vi "simulate_3d_spiral.vi"(8 "error in (no error)":errorcluster, 10 "open fp?":bool, 11 "TrajectoryMH100122AODRAPS in":refnum<class "TrajectoryMH100122AODRAPS.lvclass">) -> (0 "error out":errorcluster, 3 "TrajectoryMH100122AODRAPS out":refnum<class "TrajectoryMH100122AODRAPS.lvclass">)   [LabVIEW 2010, in "TrajectoryMH100122AODRAPS.lvclass"]
uses:
  TrajectoryMH100122AODRAPS.lvclass
  <vilib>/Math Plots/3D Math Plots/3D Scatter/3D Scatter XCtrl/3D Scatter.xctl
  <vilib>/Math Plots/3D Math Plots/3D Scatter/3D Scatter Datatype/Public/Plot Helper (Vector).vi
  <vilib>/Math Plots/3D Math Plots/3D Scatter/3D Scatter Datatype/3D Scatter Datatype.lvclass
panel:
  out "3D plot":refnum<class "3D Plot Datatype.lvclass">[](xcontrol)
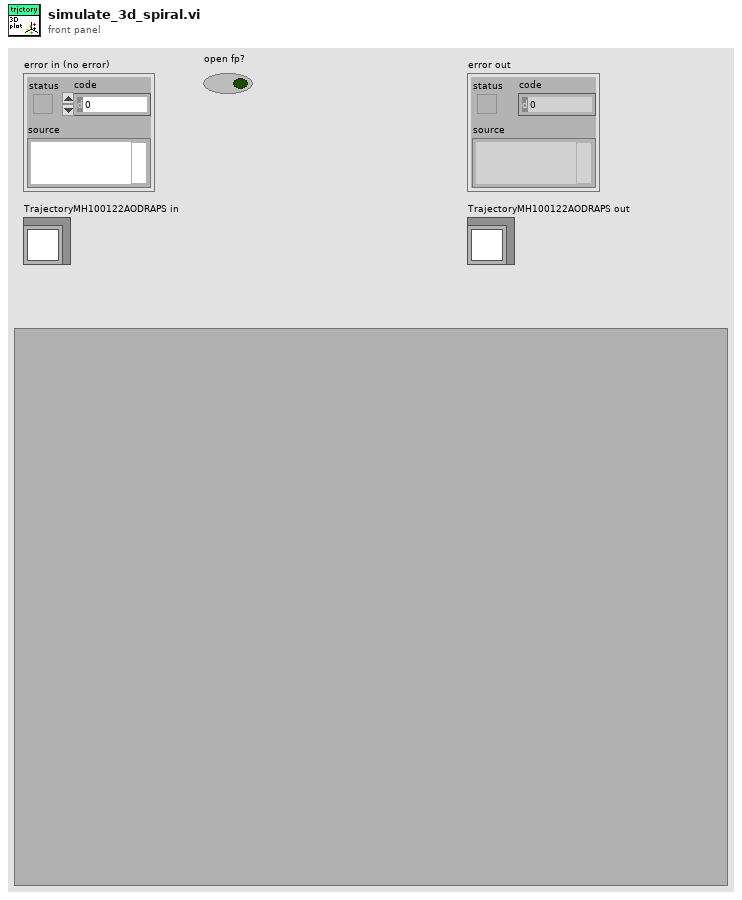
[diagram p1: front panel]
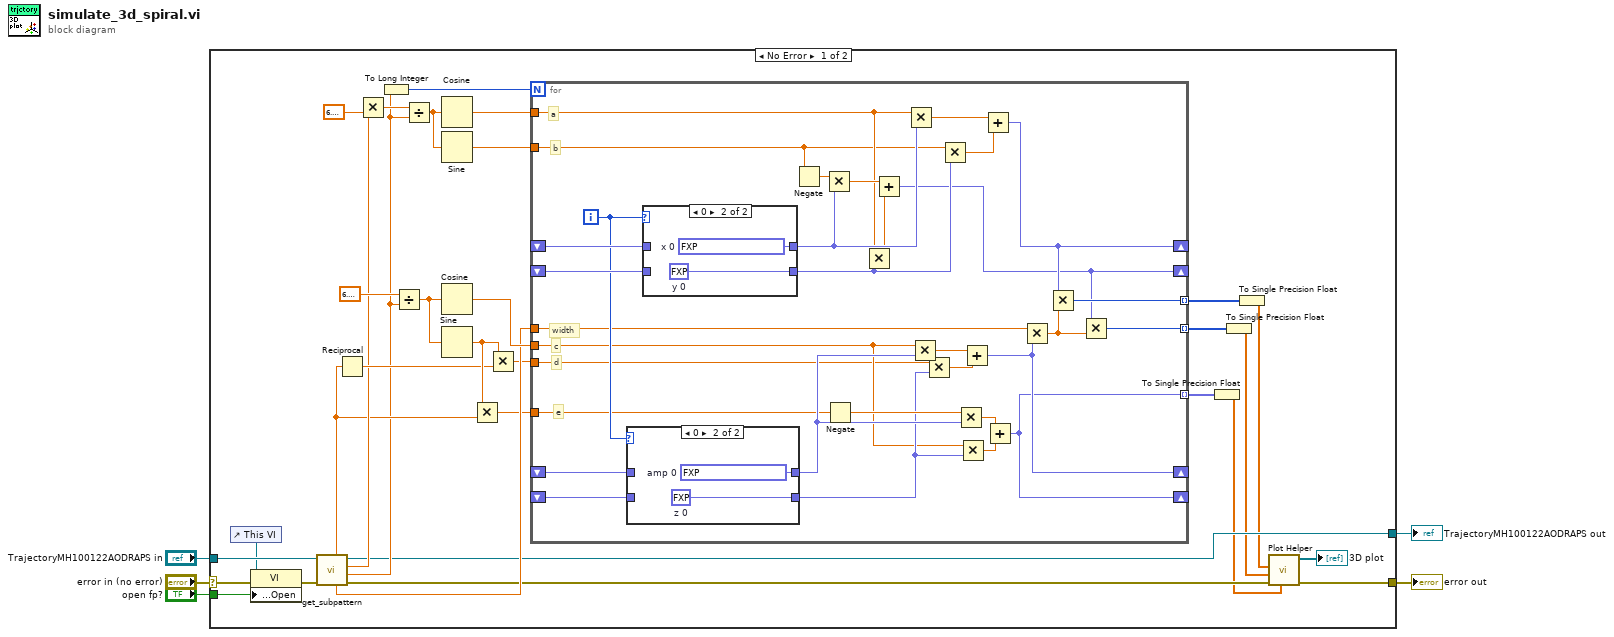
[diagram p0: block diagram]
diagram:
  n1 = case shown="No Error" "error in (no error)" {
    selector: "error in (no error)" -> [w9 w79]
    tunnel: [w18 w79] -> w4
    tunnel: [w17 w78] -> w2
    tunnel: "TrajectoryMH100122AODRAPS in" -> [w37 w78]
    tunnel: "open fp?" -> [w6 _]
    frame No Error {
      n2 = control-ref of="This VI"() -> (w7:refnum<vi>)
      n3 = property class="VI"(reference=w7, error in=w9, "Front Panel.Open"=w6) -> (error out=w8:errorcluster)  [unwired: 1 out]
      n4 = call-dynamic "get_subpattern.vi"("error in (no error)"=w8, "TrajectoryMH100122AODRAPS in"=w37) -> ("error out"=w19:errorcluster, "number of iteration points"=w27:dbl, "winding number"=w29:dbl, "TrajectoryMH100122AODRAPS out"=w17:refnum<class "TrajectoryMH100122AODRAPS.lvclass">, "diameter"=w22:dbl, "height"=w28:dbl)  [unwired: 4 in]
      n5 = Reciprocal(x=w28) -> (1/x=w33:dbl)
      n6 = Multiply(x=w29, y=6.283185307179586) -> (x*y=w31:dbl)
      n7 = To Long Integer(number=w27) -> (32bit integer=w26:i32)
      n8 = Divide(x=6.283185307179586, y=w27) -> (x/y=w36:dbl)
      n9 = Divide(x=w31, y=w27) -> (x/y=w32:dbl)
      n10 = Cosine(x=w32) -> (cos(x)=w25:dbl)
      n11 = Sine(x=w32) -> (sin(x)=w24:dbl)
      n12 = Cosine(x=w36) -> (cos(x)=w23:dbl)
      n13 = Sine(x=w36) -> (sin(x)=w34:dbl)
      n14 = Multiply(x=w34, y=w28) -> (x*y=w20:dbl)
      n15 = Multiply(x=w34, y=w33) -> (x*y=w21:dbl)
      n16 = for {
        N: w26 -> [_]
        shift-right: [w50] -> _
        shift-left: _ -> [w62]
        shift-right: [w48] -> _
        shift-left: _ -> [w61]
        shift-right: [w47] -> _
        shift-left: _ -> [w57]
        shift-right: [w44] -> _
        shift-left: _ -> [w51]
        tunnel: [w49] -> w16 mode=indexing
        tunnel: [w45] -> w14 mode=indexing
        tunnel: [w44] -> w15 mode=indexing
        tunnel: w25 -> [w43]
        tunnel: w24 -> [w42]
        tunnel: w23 -> [w41]
        tunnel: w22 -> [w40]
        tunnel: w21 -> [w39]
        tunnel: w20 -> [w38]
        i -> [w60]
        # "e"
        # "width"
        # "b"
        # "a"
        # "c"
        # "d"
        n17 = case shown="0" w60 {
          tunnel: [w71 w73] -> w54
          tunnel: [w70 w72] -> w55
          tunnel: w57 -> [w70 _]
          tunnel: w51 -> [w71 _]
          frame Default {
          }
          frame 0 {
            w72 = fxp<+/-,16,1> 0.999969482421875  # amp 0
            w73 = fxp<+/-,16,8> 0.0  # z 0
          }
        }
        n18 = case shown="0" w60 {
          tunnel: [w74 w77] -> w65
          tunnel: [w75 w76] -> w66
          tunnel: w62 -> [w75 _]
          tunnel: w61 -> [w74 _]
          frame Default {
          }
          frame 0 {
            w76 = fxp<+/-,16,1> 0.999969482421875  # x 0
            w77 = fxp<+/-,16,1> 0.0  # y 0
          }
        }
        n19 = Negate(x=w42) -> (-x=w67:dbl)
        n20 = Multiply(x=w67, y=w66) -> (x*y=w63:dbl)
        n21 = Negate(x=w38) -> (-x=w56:dbl)
        n22 = Multiply(x=w43, y=w65) -> (x*y=w64:dbl)
        n23 = Add(x=w63, y=w64) -> (x+y=w48:fxp<+/-,16,1>)
        n24 = Multiply(x=w43, y=w66) -> (x*y=w69:dbl)
        n25 = Multiply(x=w41, y=w55) -> (x*y=w59:dbl)
        n26 = Multiply(x=w39, y=w54) -> (x*y=w58:dbl)
        n27 = Multiply(x=w42, y=w65) -> (x*y=w68:dbl)
        n28 = Multiply(x=w56, y=w55) -> (x*y=w53:dbl)
        n29 = Multiply(x=w41, y=w54) -> (x*y=w52:dbl)
        n30 = Add(x=w59, y=w58) -> (x+y=w47:fxp<+/-,16,1>)
        n31 = Add(x=w69, y=w68) -> (x+y=w50:fxp<+/-,16,1>)
        n32 = Add(x=w53, y=w52) -> (x+y=w44:fxp<+/-,32,16>)
        n33 = Multiply(x=w40, y=w47) -> (x*y=w46:dbl)
        n34 = Multiply(x=w50, y=w46) -> (x*y=w49:i32)
        n35 = Multiply(x=w48, y=w46) -> (x*y=w45:i32)
      }
      n36 = To Single Precision Float(number=w15) -> (single precision float=w11:sgl[])
      n37 = To Single Precision Float(number=w14) -> (single precision float=w12:sgl[])
      n38 = To Single Precision Float(number=w16) -> (single precision float=w13:sgl[])
      n39 = call-poly <vilib>:"Plot Helper.vi"("z vector"=w11, "error in (no error)"=w19, "y vector"=w12, "x vector"=w13) -> ("error out"=w18:errorcluster, "3D Plot lvclass Array out"=→"3D plot":refnum<class "3D Plot Datatype.lvclass">[])  [unwired: 2 in, 4 out]
    }
    frame Error {
    }
  }
  "error out" <- w4
  "TrajectoryMH100122AODRAPS out" <- w2
